vi "Pause measurements.vi"(8 "error in (no error)":errorcluster, 10 "Pause":bool, 11 "Mag Lab Measure Controller in":refnum<class "Mag Lab Measure Controller.lvclass">) -> (0 "error out":errorcluster, 3 "Mag Lab Measure Controller out":refnum<class "Mag Lab Measure Controller.lvclass">)   [LabVIEW 2015, in "Mag Lab Measure Controller.lvclass"]
uses:
  Mag Lab Measure Controller.lvclass
  Mag Lab Measure Controller.lvclass/Mag Lab Measure Controller.ctl
  Mag Lab Root/Mag Lab Root.lvclass/Mag Lab Root.ctl
  Mag Lab Measurement/Mag Lab Measurement.lvclass/Mag Lab Measurement.ctl
  Mag Lab Root/Mag Lab Root.lvclass
  Mag Lab Measurement/Mag Lab Measurement.lvclass
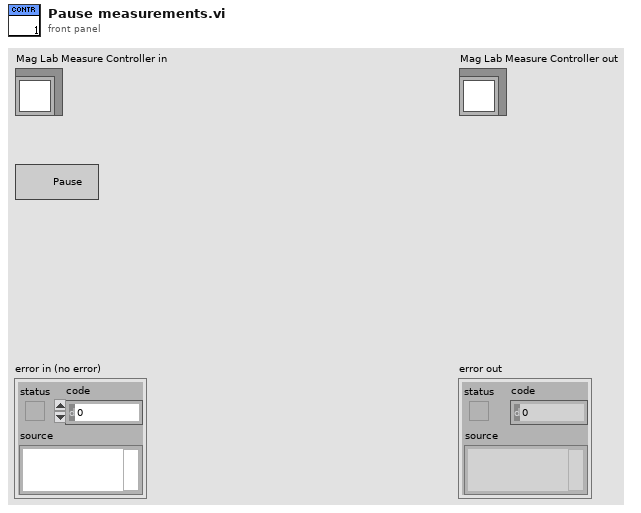
[diagram p1: front panel]
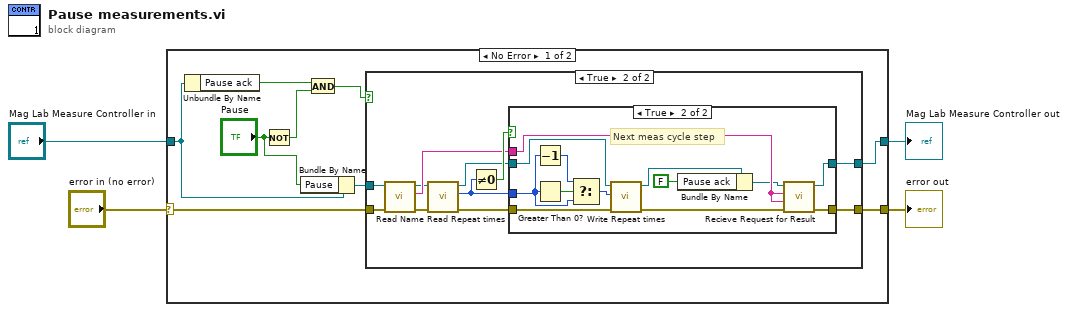
[diagram p0: block diagram]
diagram:
  n1 = case shown="No Error" "error in (no error)" {
    selector: "error in (no error)" -> [w9 w43]
    tunnel: [w8 w43] -> w3
    tunnel: "Mag Lab Measure Controller in" -> [w7 w42]
    tunnel: [w5 w42] -> w1
    frame No Error {
      n2 = Unbundle By Name(w7) -> ("Pause ack"=w13:bool)
      n3 = Not(x="Pause") -> (.not. x?=w10:bool)
      n4 = Bundle By Name(cluster=w7, "Pause"="Pause") -> (w6:refnum<class "Mag Lab Measure Controller.lvclass">)
      n5 = And(x=w13, y=w10) -> (x .and. y?=w11:bool)
      n6 = case shown="True" w11 {
        tunnel: w9 -> [w15 w21]
        tunnel: [w15 w20] -> w8
        tunnel: w6 -> [w14 w19]
        tunnel: [w14 w16] -> w5
        frame False {
        }
        frame True {
          n7 = call "Read Name.vi"("error in (no error)"=w21, "Mag Lab Root in"=w19) -> ("error out"=w23:errorcluster, "Name"=w22:string, "Mag Lab Root out"=w18:refnum<class "Mag Lab Measure Controller.lvclass">)  [unwired: 7 in]
          n8 = call "Read Repeat times.vi"("error in (no error)"=w23, "Mag Lab Measurement in"=w18) -> ("error out"=w25:errorcluster, "Repeat times"=w26:i32, "Mag Lab Measurement out"=w17:refnum<class "Mag Lab Measure Controller.lvclass">)  [unwired: 7 in]
          n9 = Not Equal To 0?(x=w26) -> (x != 0?=w24:bool)
          n10 = case shown="True" w24 {
            tunnel: w25 -> [w28 w36]
            tunnel: w22 -> [_ w41]
            tunnel: w26 -> [_ w38]
            tunnel: [w28 w34] -> w20
            tunnel: w17 -> [w27 w33]
            tunnel: [w27 w29] -> w16
            frame False {
              # "Measurements finished"
            }
            frame True {
              # "Next meas cycle step"
              n11 = Decrement(x=w38) -> (x-1=w39:i32)
              n12 = Greater Than 0?(x=w38) -> (x > 0?=w40:bool)
              n13 = Select(t=w39, s=w40, f=w38) -> (s? t:f=w37:i32)
              n14 = call "Write Repeat times.vi"("error in (no error)"=w36, "Repeat times"=w37, "Mag Lab Measurement in"=w33) -> ("error out"=w35:errorcluster, "Mag Lab Measurement out"=w32:refnum<class "Mag Lab Measure Controller.lvclass">)  [unwired: 7 in]
              n15 = Bundle By Name(cluster=w32, "Pause ack"=FALSE) -> (w31:refnum<class "Mag Lab Measure Controller.lvclass">)
              n16 = call-dynamic "Recieve Request for Result.vi"("error in (no error)"=w35, "Requestor"=w41, "Requestee"=w41, "Mag Lab Measure Controller in"=w31) -> ("error out"=w34:errorcluster, "Mag Lab Measure Controller out"=w29:refnum<class "Mag Lab Measure Controller.lvclass">)  [unwired: 6 in]
            }
          }
        }
      }
    }
    frame Error {
    }
  }
  "error out" <- w3
  "Mag Lab Measure Controller out" <- w1
